vi "Stimulus XCtl Test.vi"(0 "StimChans In":T29[](array[typedef])=[{"Waveform"={"Type"=enum."Tone", "Tone"={"Frequency (kHz)"=8.0, "Phase (cycles)"=0.0, "Random phase"=TRUE}, "Pulse Train"={"Pulse width (us)"=0.0, "Pulse rate (Hz)"=0.0, "Gap (ms)"=0.0, "Polarity"=enum."POS", "PT State"={"Template"=[], "Nperiod"=0, "Index"=0, "Pulse Rate (Hz)"=0.0, "Phase (cycles)"=0.0, "Noff"=0}, "Asynch"=FALSE}, "Noise"={"Properties"={"InvFilt"=FALSE, "Aweight"=FALSE, "Seed"=0, "Tokens"=0}, "Data"={"TokenNum"=0}}, "File"={"Filename"=path "", "Signal"=[], "Channel"=0}, "FMSweep"={"Rate (oct/s)"=0.0, "Fmin (Hz)"=0.0, "Fmax (Hz)"=0.0, "Ramp (ms)"=0.0, "Linear"=FALSE}, "Chirp Train"={"Params"={"Fmin (kHz)"=4.0, "Fmax (kHz)"=64.0, "Compensate"=FALSE, "Duration (ms)"=2.0}, "Data"={"WF"=[]}}, "Complex Tone"={"Params"={"F0 (Hz)"=0.0, "Band"={"Flow (Hz)"=0.0, "Fhigh (Hz)"=0.0}, "Phase"=enum."Cosine", "Min F0 (Hz)"=0.0, "Max F0 (Hz)"=0.0, "ContinRandPhase"=FALSE, "Max peak factor"=inf, "Max mod depth"=2.0, "MinHarmNum"=0, "MaxHarmNum"=0, "Level Mode"=enum."per component"}, "Data"={"Ncomp"=0, "MinHarm"=0, "Phase"=[], "Amplitude"=[], "Npts/frame"=0, "Last F0"=0.0, "Fmin"=0.0, "Fmax"=0.0, "Lslope"=0.0, "randphase"=FALSE, "overall rms"=FALSE}}, "FM"={"Carrier (kHz)"=0.0, "ModRate (Hz)"=0.0, "Depth (Hz)"=0.0, "Phase (cycles)"=0.0}, "Vowel"={"Freqs"="", "Set level"=enum."Total", "Freq"=[], "weights"=[]}}, "Filter"={"Type"=enum."OFF", "CF (kHz)"=0.0, "BW (kHz)"=0.0, "Cascade"=FALSE, "Quadrature"=FALSE, "Scale Factor"=0.0, "Stages"=[], "Class"=enum."Elliptic", "Order"=0, "BWUnits"=enum."Linear"}, "Burst"={"Active"=FALSE, "Delay (ms)"=0.0, "Duration (ms)"=0.0, "Ramp (ms)"=0.0, "Rate (Hz)"=0.0, "Trepeat (ms)"=0.0, "Repeat"=FALSE}, "Level"={"Level"=0.0, "Units"=enum."dB atten", "Max"=0.0, "Data"={"Multiplier"=0.0, "Cal File"=path "", "Cal"={"Freq (Hz)"=[], "Mag (dB SPL)"=[], "Phase (deg)"=[]}, "audiogram"=path ""}}, "Name"="Ch1", "Advanced"={"AltPol"=FALSE, "Var"="", "Expr"=""}, "SAM"={"Active"=FALSE, "Frequency (Hz)"=0.0, "Depth"=0.0, "Init Phase (cycles)"=0.0, "phase (degrees)"=0.0, "Asynch"=FALSE}, "Destination"={"Name"="Right", "Num"=0}}, {"Waveform"={"Type"=enum."Tone", "Tone"={"Frequency (kHz)"=8.0, "Phase (cycles)"=0.0, "Random phase"=FALSE}, "Pulse Train"={"Pulse width (us)"=0.0, "Pulse rate (Hz)"=0.0, "Gap (ms)"=0.0, "Polarity"=enum."POS", "PT State"={"Template"=[], "Nperiod"=0, "Index"=0, "Pulse Rate (Hz)"=0.0, "Phase (cycles)"=0.0, "Noff"=0}, "Asynch"=FALSE}, "Noise"={"Properties"={"InvFilt"=FALSE, "Aweight"=FALSE, "Seed"=0, "Tokens"=0}, "Data"={"TokenNum"=0}}, "File"={"Filename"=path "", "Signal"=[], "Channel"=0}, "FMSweep"={"Rate (oct/s)"=0.0, "Fmin (Hz)"=0.0, "Fmax (Hz)"=0.0, "Ramp (ms)"=0.0, "Linear"=FALSE}, "Chirp Train"={"Params"={"Fmin (kHz)"=4.0, "Fmax (kHz)"=64.0, "Compensate"=FALSE, "Duration (ms)"=2.0}, "Data"={"WF"=[]}}, "Complex Tone"={"Params"={"F0 (Hz)"=0.0, "Band"={"Flow (Hz)"=0.0, "Fhigh (Hz)"=0.0}, "Phase"=enum."Cosine", "Min F0 (Hz)"=0.0, "Max F0 (Hz)"=0.0, "ContinRandPhase"=FALSE, "Max peak factor"=inf, "Max mod depth"=2.0, "MinHarmNum"=0, "MaxHarmNum"=0, "Level Mode"=enum."per component"}, "Data"={"Ncomp"=0, "MinHarm"=0, "Phase"=[], "Amplitude"=[], "Npts/frame"=0, "Last F0"=0.0, "Fmin"=0.0, "Fmax"=0.0, "Lslope"=0.0, "randphase"=FALSE, "overall rms"=FALSE}}, "FM"={"Carrier (kHz)"=0.0, "ModRate (Hz)"=0.0, "Depth (Hz)"=0.0, "Phase (cycles)"=0.0}, "Vowel"={"Freqs"="", "Set level"=enum."Total", "Freq"=[], "weights"=[]}}, "Filter"={"Type"=enum."OFF", "CF (kHz)"=0.0, "BW (kHz)"=0.0, "Cascade"=FALSE, "Quadrature"=FALSE, "Scale Factor"=0.0, "Stages"=[], "Class"=enum."Elliptic", "Order"=0, "BWUnits"=enum."Linear"}, "Burst"={"Active"=FALSE, "Delay (ms)"=0.0, "Duration (ms)"=0.0, "Ramp (ms)"=0.0, "Rate (Hz)"=0.0, "Trepeat (ms)"=0.0, "Repeat"=FALSE}, "Level"={"Level"=0.0, "Units"=enum."dB atten", "Max"=0.0, "Data"={"Multiplier"=0.0, "Cal File"=path "", "Cal"={"Freq (Hz)"=[], "Mag (dB SPL)"=[], "Phase (deg)"=[]}, "audiogram"=path ""}}, "Name"="Ch2", "Advanced"={"AltPol"=FALSE, "Var"="", "Expr"=""}, "SAM"={"Active"=FALSE, "Frequency (Hz)"=0.0, "Depth"=0.0, "Init Phase (cycles)"=0.0, "phase (degrees)"=0.0, "Asynch"=FALSE}, "Destination"={"Name"="Left", "Num"=1}}] {"Filter"."Stages"."IIR Filter"."Forward Coefficients" format="%.4f"; "Filter"."Stages"."IIR Filter"."Reverse Coefficients" format="%.4f"}, 1 "Folder":path=path "D:/Data/XYZ DATA/XYZ999") -> ()   [LabVIEW 2015]
uses:
  XControls/Stimulus Channel (G3)/Full Stimulus Channel Data.ctl
  XControls/Waveform XControls/Waveform (G3)/Waveform Data.ctl
  Waveform VIs/Waveform Enum (V3).ctl
  XControls/Waveform XControls/Tone (G3)/Tone.Properties.ctl
  Waveform VIs/Pulse Train VIs/Pulse Train Params.ctl
  Waveform VIs/Pulse Train VIs/Pulse Polarity.ctl
  Waveform VIs/Pulse Train VIs/PT-Continuous State.ctl
  Waveform VIs/Noise VIs/Noise (G3).ctl
  Waveform VIs/Noise VIs/Noise (G3).Properties.ctl
  Waveform VIs/Noise VIs/Noise (G3).Data.ctl
  Waveform VIs/File VIs/StimFile-Params.ctl
  Waveform VIs/FM Sweep VIs/FM Sweep Params.ctl
  Waveform VIs/Chirp Train VIs/Chirp Train.ctl
  Waveform VIs/Chirp Train VIs/Chirp Train Params.ctl
  Waveform VIs/Complex Tone VIs/CT-Params.ctl
  Waveform VIs/Complex Tone VIs/CT-Phase Enum.ctl
  Waveform VIs/Complex Tone VIs/CT-Runtime Data.ctl
  XControls/Waveform XControls/FM Tone/Data.ctl
  XControls/Waveform XControls/Vowel/Vowel.Properties.ctl
  XControls/Filter (G3)/Filter Data.ctl
  XControls/Filter (G3)/Filter Type.ctl
  Filter VIs/Filter-Bandwidth Units.ctl
  Controls/Burst XCtl/Burst Data.ctl
  XControls/Level (G3)/Level Data.ctl
  XControls/Level (G3)/Level Units (G3).ctl
  XControls/Advanced Options (G3)/Advanced Options (G3).ctl
  Modulation VIs/SAM VIs/SAM Params.ctl
  Typedefs/Destination.ctl
  XControls/Stimulus Channel (G3)/Stimulus Channel (G3).xctl
  XControls/Waveform XControls/Waveform (G3)/Waveform (G3).xctl
  XControls/Filter (G3)/Filter (G3).xctl
  Controls/Burst XCtl/Burst Control.xctl
  XControls/Level (G3)/Level (G3).xctl
  XControls/Advanced Options (G3)/Advanced Options (G3).xctl
  XControls/Waveform XControls/Tone (G3)/Tone (G3).xctl
  XControls/Waveform XControls/FM Tone/FM Tone.xctl
  XControls/Waveform XControls/Vowel/Vowel.xctl
panel:
  in  "Drag from":i32
  in  "StimChan":T28(xcontrol)
  out "exit signal":bool
  in  "Delete":bool
  in  "Insert":bool
  in  "Apply":bool
  in  "Channels":i32[](listbox)
  # "Right Primary"
  # "Right Primary"
  # "Laser1"
  # "Right Primary"
  # "Right Primary"
  # "Laser2"
  # "Right Primary"
  # "Shutter"
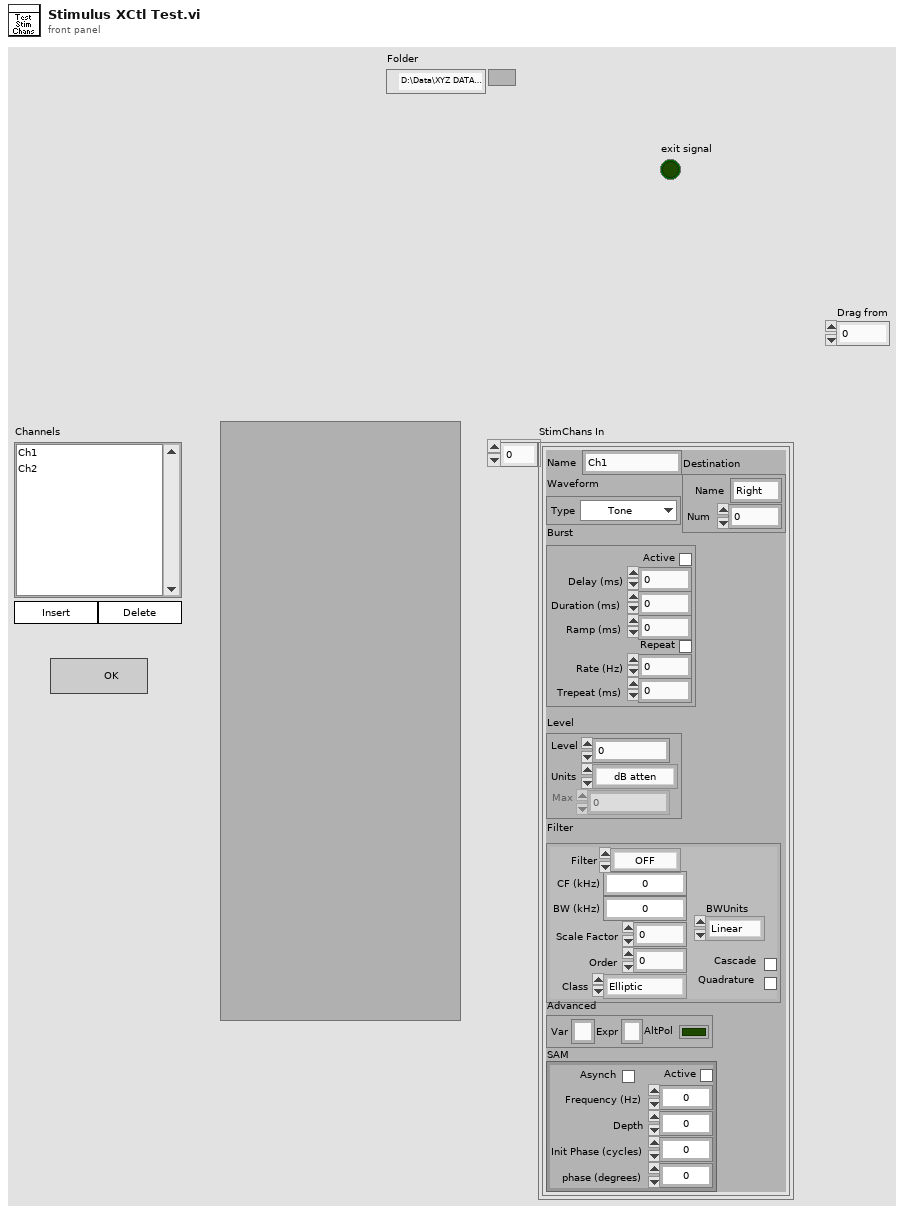
[diagram p1: front panel]
types:
  T1 = typedef "Waveform (G3).xctl/Waveform Data.ctl" = cluster{"Type":T2, "Tone":T3, "Pulse Train":T4, "Noise":T7, "File":T10, "FMSweep":T11, "Chirp Train":T12, "Complex Tone":cluster{"Params":T14, "Data":T16}, "FM":T17, "Vowel":T18}
  T2 = typedef "Waveform Enum (V3).ctl" = enum16{"OFF", "Tone", "Noise", "Pulse Train", "File", "FM Sweep", "Chirp Train", "Complex Tone", "FM Tone", "Vowel"}
  T3 = typedef "Tone (G3).xctl/Tone.Properties.ctl" = cluster{"Frequency (kHz)":dbl, "Phase (cycles)":dbl, "Random phase":bool}
  T4 = typedef "Pulse Train Params.ctl" = cluster{"Pulse width (us)":dbl, "Pulse rate (Hz)":dbl, "Gap (ms)":dbl, "Polarity":T5, "PT State":T6, "Asynch":bool}
  T5 = typedef "Pulse Polarity.ctl" = enum16{"POS", "NEG", "POS-NEG", "NEG-POS"}
  T6 = typedef "PT-Continuous State.ctl" = cluster{"Template":dbl[], "Nperiod":i32, "Index":i32, "Pulse Rate (Hz)":dbl, "Phase (cycles)":dbl, "Noff":i32}
  T7 = typedef "Noise (G3).ctl" = cluster{"Properties":T8, "Data":T9}
  T8 = typedef "Noise (G3).Properties.ctl" = cluster{"InvFilt":bool, "Aweight":bool, "Seed":i32, "Tokens":i32}
  T9 = typedef "Noise (G3).Data.ctl" = cluster{"TokenNum":i32}
  T10 = typedef "StimFile-Params.ctl" = cluster{"Filename":path, "Signal":dbl[], "Channel":i32}
  T11 = typedef "FM Sweep Params.ctl" = cluster{"Rate (oct/s)":dbl, "Fmin (Hz)":dbl, "Fmax (Hz)":dbl, "Ramp (ms)":dbl, "Linear":bool}
  T12 = typedef "Chirp Train.ctl" = cluster{"Params":T13, "Data":cluster{"WF":dbl[]}}
  T13 = typedef "Chirp Train Params.ctl" = cluster{"Fmin (kHz)":dbl, "Fmax (kHz)":dbl, "Compensate":bool, "Duration (ms)":dbl}
  T14 = typedef "CT-Params.ctl" = cluster{"F0 (Hz)":dbl, "Band":cluster{"Flow (Hz)":dbl, "Fhigh (Hz)":dbl}, "Phase":T15, "Min F0 (Hz)":dbl, "Max F0 (Hz)":dbl, "ContinRandPhase":bool, "Max peak factor":dbl, "Max mod depth":dbl, "MinHarmNum":i32, "MaxHarmNum":i32, "Level Mode":enum16{"per component", "overall rms"}}
  T15 = typedef "CT-Phase Enum.ctl" = enum16{"Cosine", "Random", "Alternating"}
  T16 = typedef "CT-Runtime Data.ctl" = cluster{"Ncomp":i32, "MinHarm":i32, "Phase":dbl[], "Amplitude":dbl[], "Npts/frame":i32, "Last F0":dbl, "Fmin":dbl, "Fmax":dbl, "Lslope":dbl, "randphase":bool, "overall rms":bool}
  T17 = typedef "FM Tone.xctl/Data.ctl" = cluster{"Carrier (kHz)":dbl, "ModRate (Hz)":dbl, "Depth (Hz)":dbl, "Phase (cycles)":dbl}
  T18 = typedef "Vowel.xctl/Vowel.Properties.ctl" = cluster{"Freqs":string, "Set level":enum16{"Total", "Per component"}, "Freq":dbl[], "weights":dbl[]}
  T19 = typedef "Filter (G3).xctl/Filter Data.ctl" = cluster{"Type":T20, "CF (kHz)":dbl, "BW (kHz)":dbl, "Cascade":bool, "Quadrature":bool, "Scale Factor":dbl, "Stages":cluster{"IIR Filter":cluster{"filter structure":enum32{"IIR 2nd Order", "IIR 4th Order"}, "Reverse Coefficients":dbl[], "Forward Coefficients":dbl[]}, "State":dbl[]}[], "Class":enum16{"Elliptic", "Butterworth"}, "Order":i32, "BWUnits":T21}
  T20 = typedef "Filter (G3).xctl/Filter Type.ctl" = enum16{"OFF", "Lowpass", "Highpass", "Bandpass", "Bandstop"}
  T21 = typedef "Filter-Bandwidth Units.ctl" = enum16{"Linear", "Octaves", "Min-Max"}
  T22 = typedef "Burst Control.xctl/Burst Data.ctl" = cluster{"Active":bool, "Delay (ms)":dbl, "Duration (ms)":dbl, "Ramp (ms)":dbl, "Rate (Hz)":dbl, "Trepeat (ms)":dbl, "Repeat":bool}
  T23 = typedef "Level (G3).xctl/Level Data.ctl" = cluster{"Level":dbl, "Units":T24, "Max":dbl, "Data":cluster{"Multiplier":dbl, "Cal File":path, "Cal":cluster{"Freq (Hz)":dbl[], "Mag (dB SPL)":dbl[], "Phase (deg)":dbl[]}, "audiogram":path}}
  T24 = typedef "Level (G3).xctl/Level Units (G3).ctl" = enum16{"dB atten", "dB SPL", "dB re 1 Vrms", "dB V/Hz½", "dB SL", "mW", "Volts"}
  T25 = typedef "Advanced Options (G3).xctl/Advanced Options (G3).ctl" = cluster{"AltPol":bool, "Var":string, "Expr":string}
  T26 = typedef "SAM Params.ctl" = cluster{"Active":bool, "Frequency (Hz)":dbl, "Depth":dbl, "Init Phase (cycles)":dbl, "phase (degrees)":dbl, "Asynch":bool}
  T27 = typedef "Destination.ctl" = cluster{"Name":string, "Num":i32}
  T28 = cluster{"Waveform":T1, "Filter":T19, "Burst":T22, "Level":T23, "Name":string, "Advanced":T25, "SAM":T26, "Destination":T27}
  T29 = typedef "Stimulus Channel (G3).xctl/Full Stimulus Channel Data.ctl" = cluster{"Waveform":T1, "Filter":T19, "Burst":T22, "Level":T23, "Name":string, "Advanced":T25, "SAM":T26, "Destination":T27}
  T30 = typedef "Endpoint-Spec.ctl" = cluster{"Name":string, "Modality":T31, "Laterality":T32, "CalFile":path, "Audiogram":path, "reuse cal?":bool}
  T31 = typedef "Endpoint-Modality.ctl" = enum16{"Unspecified", "Acoustic", "Electric", "Optical"}
  T32 = typedef "Endpoint-Laterality.ctl" = enum16{"N/A", "Right", "Left"}
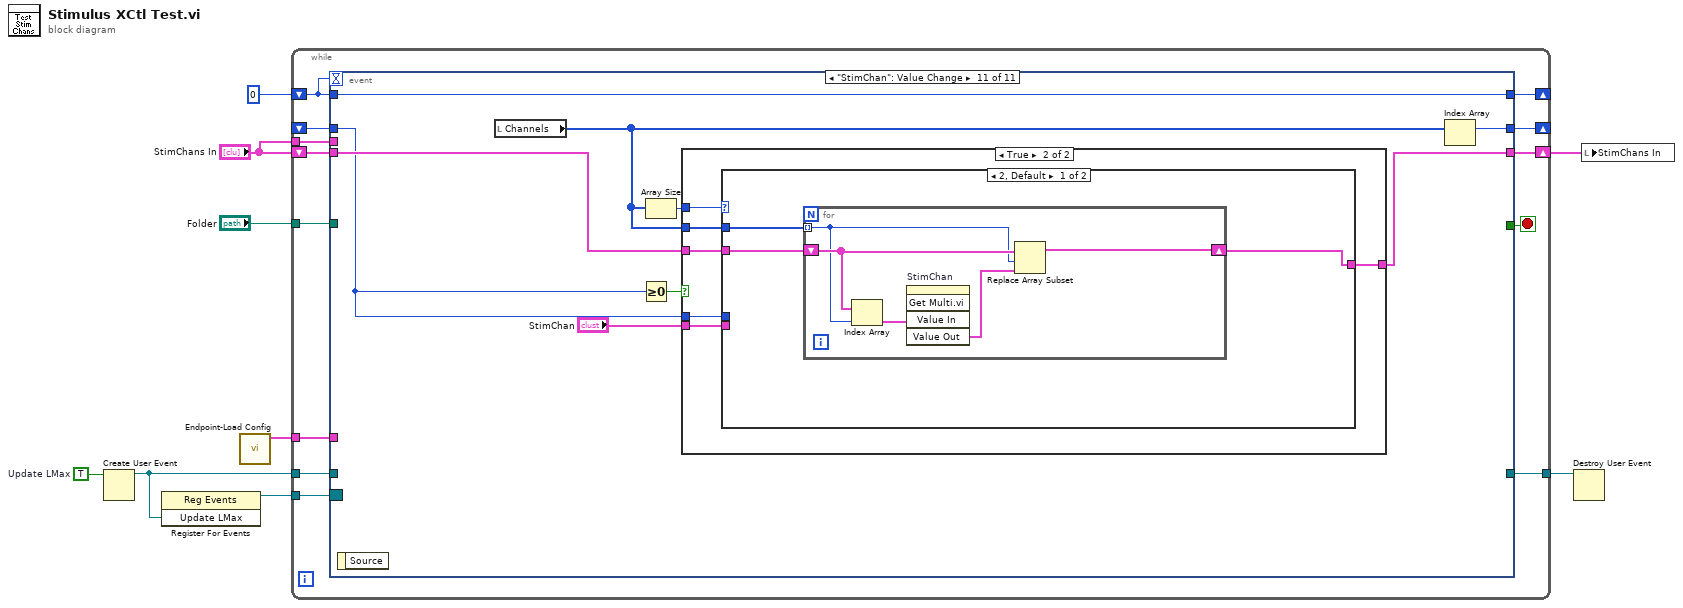
[diagram p0: block diagram]
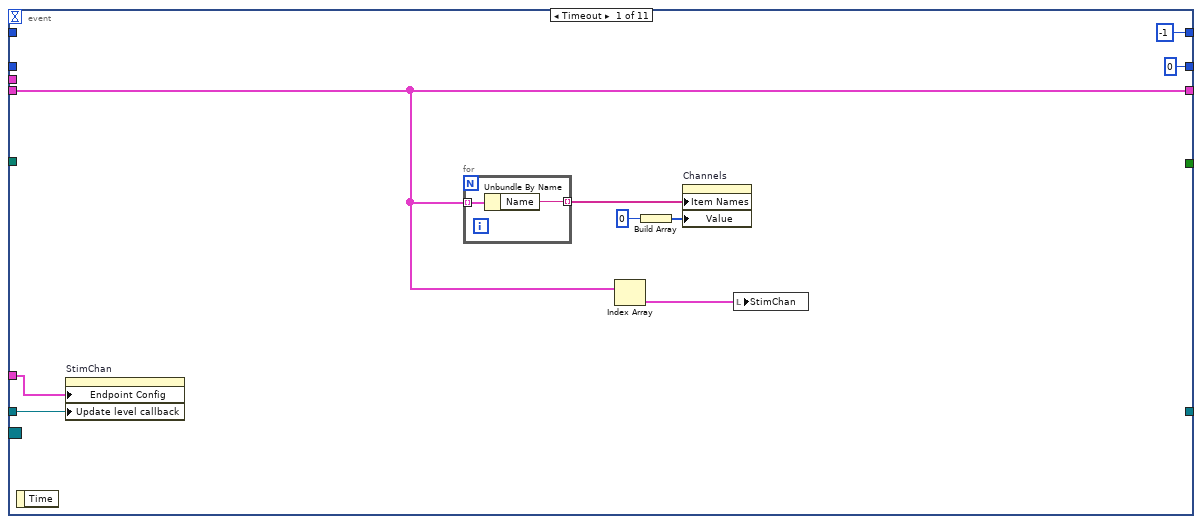
[diagram p2: hidden frame]
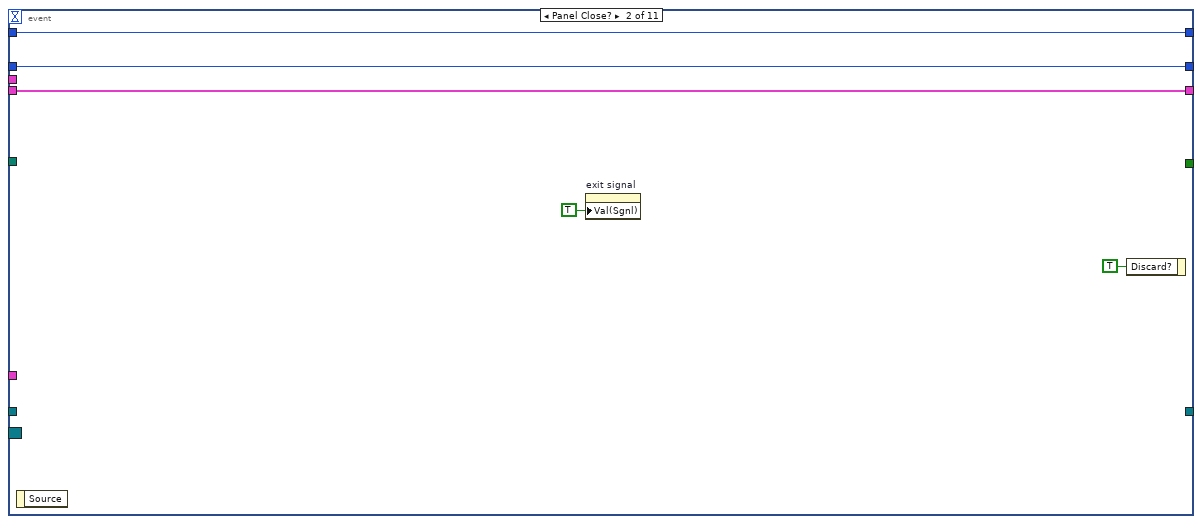
[diagram p3: hidden frame]
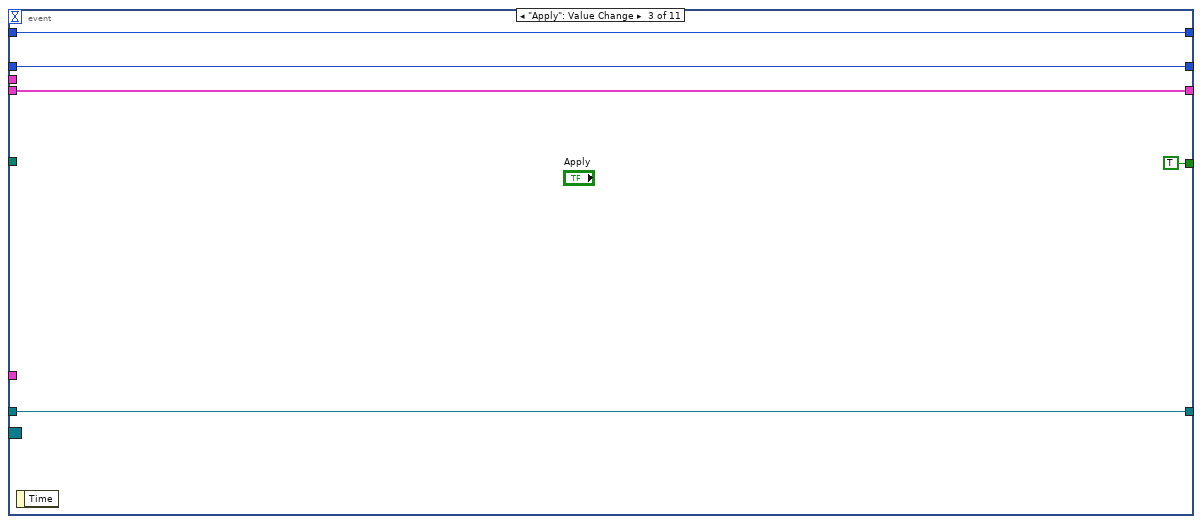
[diagram p4: hidden frame]
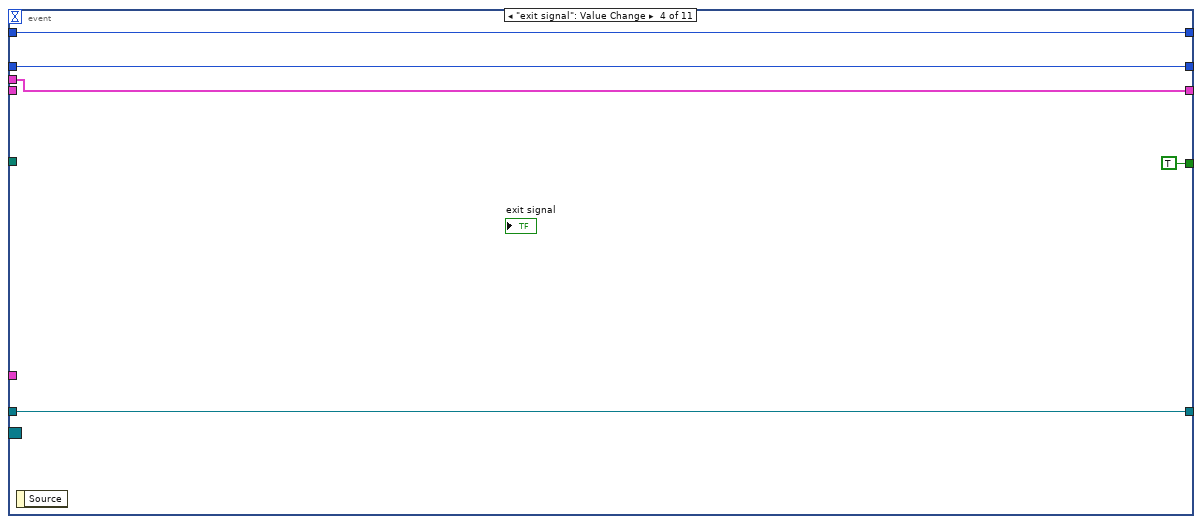
[diagram p5: hidden frame]
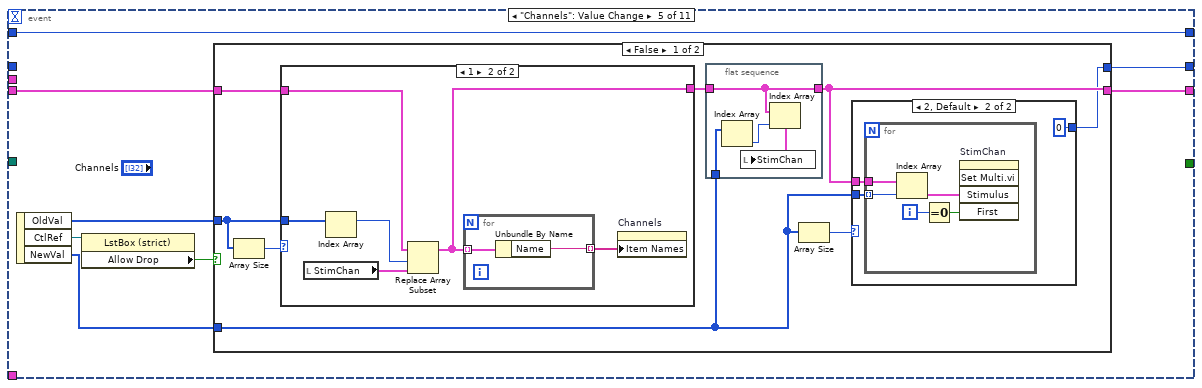
[diagram p6: hidden frame]
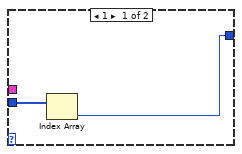
[diagram p7: hidden frame]
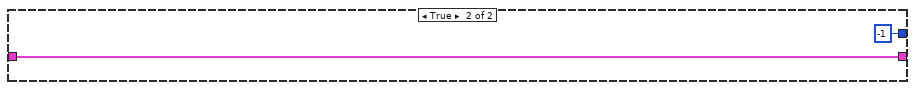
[diagram p9: hidden frame]
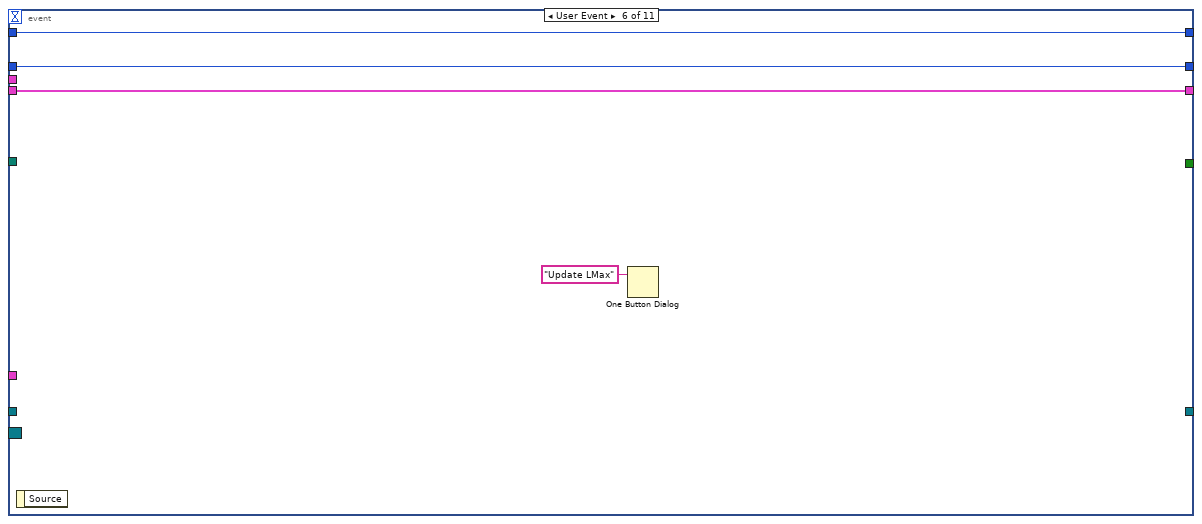
[diagram p10: hidden frame]
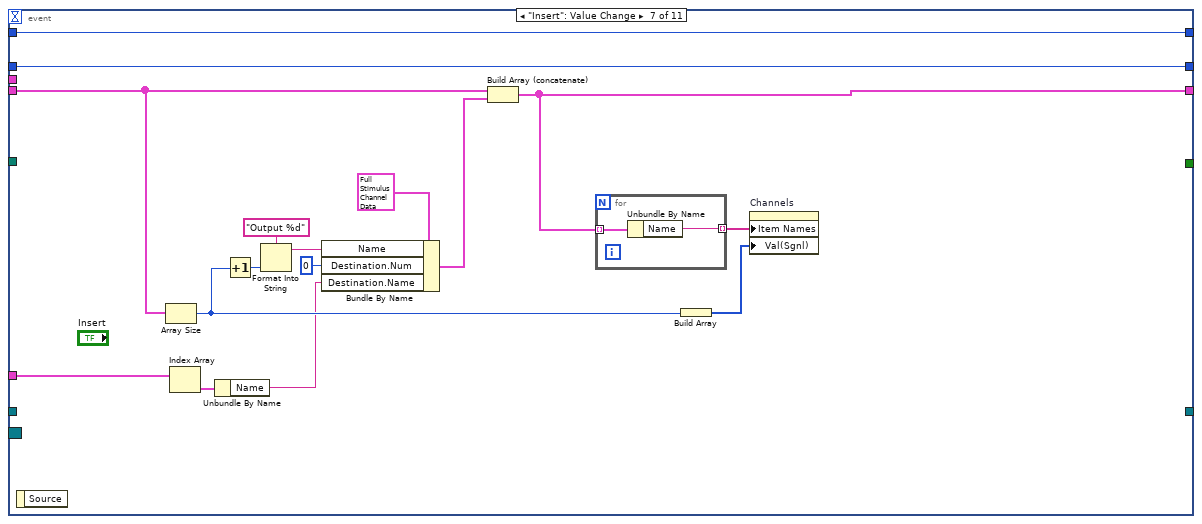
[diagram p11: hidden frame]
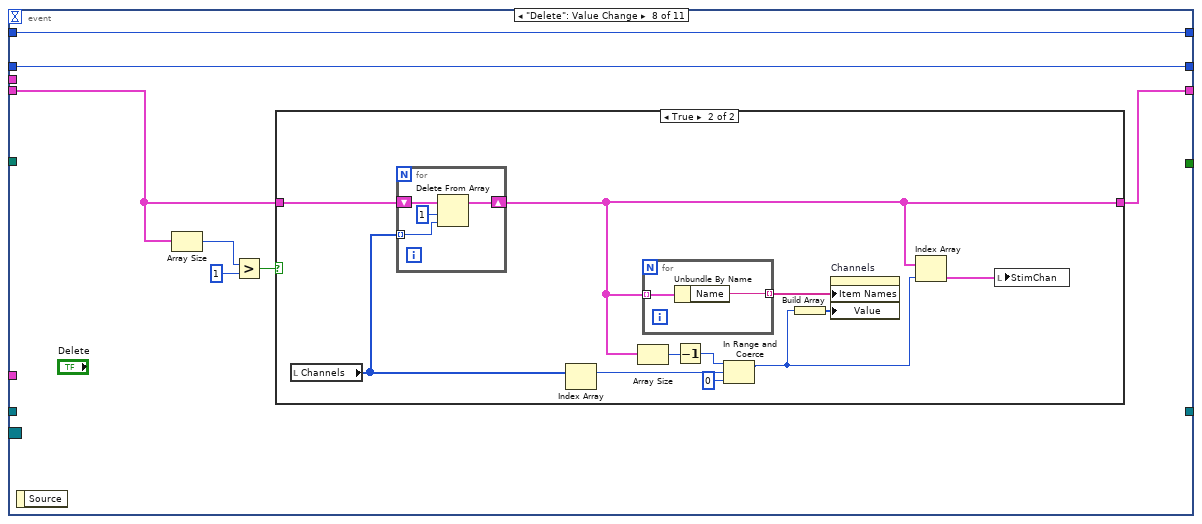
[diagram p12: hidden frame]
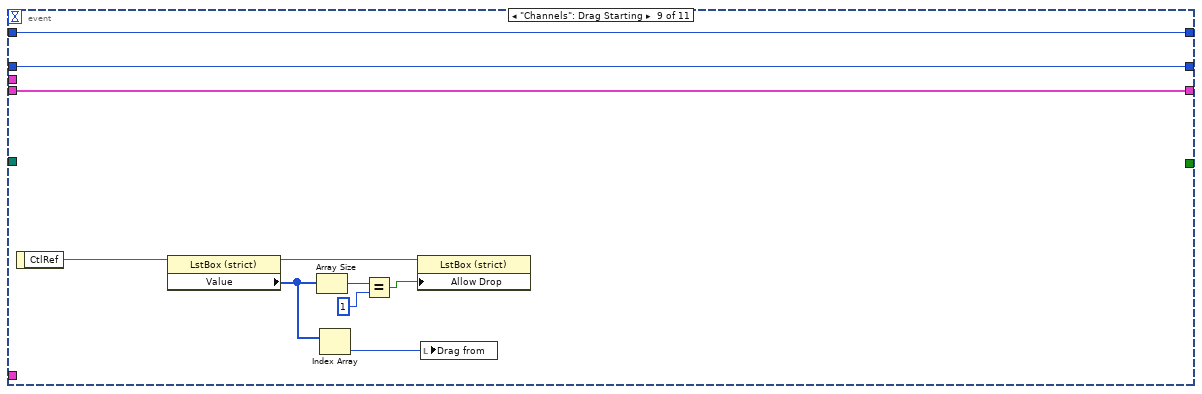
[diagram p14: hidden frame]
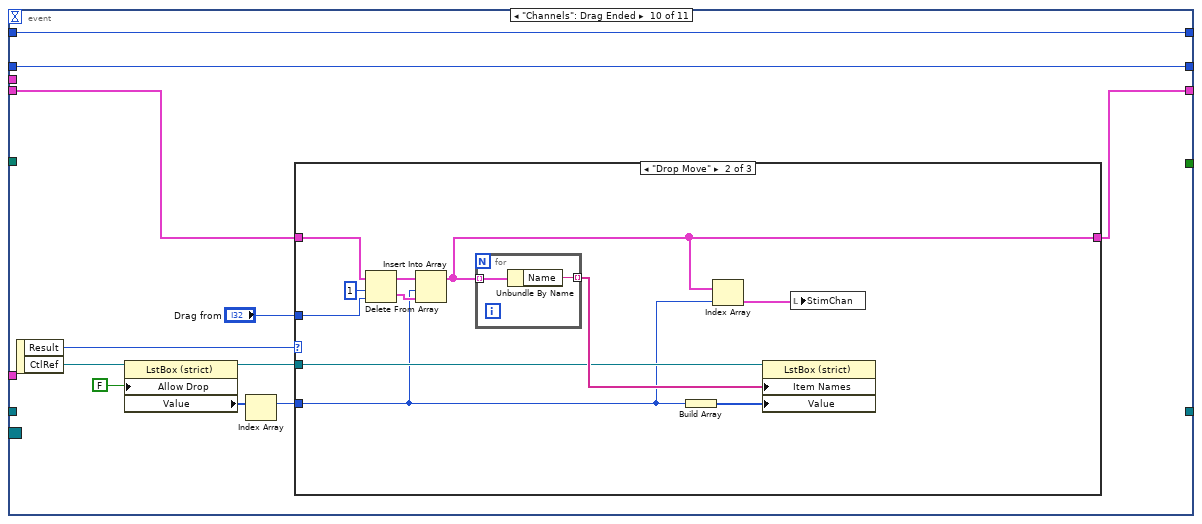
[diagram p15: hidden frame]
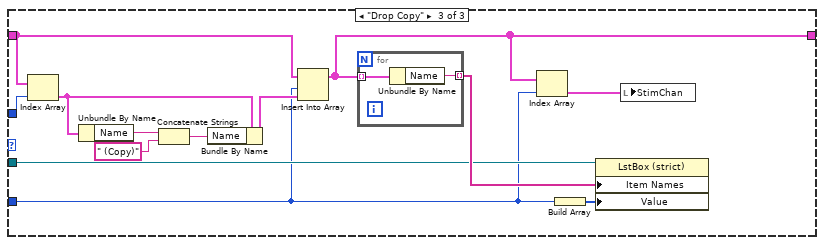
[diagram p17: hidden frame]
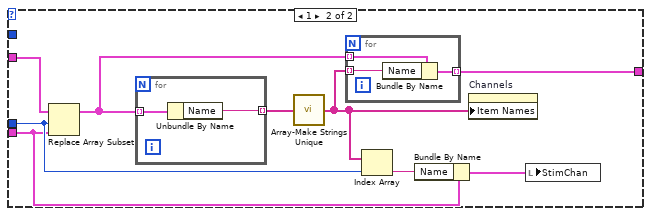
[diagram p19: hidden frame]
diagram:
  w7 = TRUE  # Update LMax
  n1 = Create User Event(user event datatype=w7) -> (user event=w5:refnum<user-event>)  [unwired: 1 in, 1 out]
  n2 = register-events(w5) -> (reference out=w6:refnum<event-registration>)  [unwired: 2 in, 1 out]
  n3 = call "Endpoint-Load Config.vi"() -> ("Endpoint Config"=w2:T30[])  [unwired: 10 in, 1 out]
  n4 = while {
    shift-right: [w22] -> _
    shift-left: 0 -> [w20]
    shift-right: [w18] -> w1
    shift-left: "StimChans In" -> [w19]
    tunnel: "StimChans In" -> [w17]
    tunnel: w6 -> [w16]
    tunnel: w5 -> [w15]
    tunnel: w2 -> [w14]
    tunnel: "Folder" -> [w13]
    shift-right: [w12] -> _
    shift-left: _ -> [w11]
    tunnel: [w10] -> w3
    stop <- w21 stop-if-true
    n5 = event shown="[10] \"StimChan\": Value Change" {
      selector: w16 -> [_ _ _ _ _ _ _ _ _ _ _]
      dyn-events: _ -> [_ _ _ _ _ _ _ _ _ _ _]
      timeout: w20 -> [_ _ _ _ _ _ _ _ _ _ _]
      tunnel: [-1 w38 w42 w47 w56 w93 w109 w118 w146 w157 w195] -> w22
      tunnel: [_ _ TRUE TRUE _ _ _ _ _ _ _] -> w21
      tunnel: w20 -> [_ w38 w42 w47 w56 w93 w109 w118 w146 w157 w195]
      tunnel: w19 -> [w27 w37 w41 _ w54 w92 w108 w115 w145 w153 w194]
      tunnel: [w27 w37 w41 w46 w53 w92 w102 w114 w145 w151 w193] -> w18
      tunnel: w17 -> [_ _ _ w46 _ _ _ _ _ _ _]
      tunnel: w15 -> [w30 _ w39 w44 _ _ _ _ _ _ _]
      tunnel: w14 -> [w31 _ _ _ _ _ w98 _ _ _ _]
      tunnel: w13 -> [_ _ _ _ _ _ _ _ _ _ _]
      tunnel: [0 ("Channels") w34 w40 w45 w49 w91 w99 w112 w144 w148 w189] -> w12
      tunnel: w11 -> [_ w34 w40 w45 _ w91 w99 w112 w144 w148 w190]
      tunnel: [_ _ w39 w44 _ _ _ _ _ _ _] -> w10
      event Timeout {
        n6 = event-data() -> ()  [unwired: 1 in, 1 out]
        n7 = property on="StimChan" class="Stimulus Channel (G3) (strict)"("Endpoint Config"=w31, "Update level callback"=w30) -> ()  [unwired: 2 in, 2 out]
        n8 = for {
          tunnel: w27 -> [w33] mode=indexing
          tunnel: [w32] -> w25 mode=indexing
          n9 = Unbundle By Name(w33) -> ("Name"=w32:string)
        }
        n10 = Index Array(array=w27) -> (element=w23:T29)  [unwired: 1 in]
        n11 = Build Array(0) -> (w24:i32[])
        n12 = property on="Channels" class="LstBox (strict)"("Item Names"=w25, "Value"=w24) -> ()  [unwired: 2 in, 2 out]
        n13 = local write "StimChan"(w23) -> ()
      }
      event Panel Close? {
        n14 = event-data() -> ()  [unwired: 1 in, 1 out]
        n15 = property on="exit signal" class="Bool (strict)"("Val(Sgnl)"=TRUE ("Value (Signaling)")) -> ()  [unwired: 2 in, 2 out]
        n16 = event-data("Discard?"=TRUE) -> ()  [unwired: 1 in, 1 out]
      }
      event "Apply": Value Change {
        n17 = event-data() -> ()  [unwired: 1 in, 1 out]
      }
      event "exit signal": Value Change {
        n18 = event-data() -> ()  [unwired: 1 in, 1 out]
      }
      event "Channels": Value Change {
        n19 = event-data() -> ("OldVal"=w55:i32[], "CtlRef"=w52:refnum<vi>, "NewVal"=w50:i32[])  [unwired: 1 in]
        n20 = property class="LstBox (strict)"(reference=w52) -> ("Allow Drop"=w51:bool)  [unwired: 1 in, 2 out]
        n21 = case shown="False" w51 {
          tunnel: w55 -> [w62 _]
          tunnel: w54 -> [w61 w89]
          tunnel: [w58 w89] -> w53
          tunnel: w50 -> [w60 _]
          tunnel: [w57 -1 ("Channels")] -> w49
          frame False {
            n22 = Array Size(array=w62) -> (size(s)=w64:i32)
            n23 = case shown="1" w64 {
              tunnel: w62 -> [_ w85]
              tunnel: [w79 w81] -> w59
              tunnel: w61 -> [w79 w80]
              frame 2, Default {
              }
              frame 1 {
                n24 = local read "StimChan"() -> (w84:T28)
                n25 = Index Array(array=w85) -> (element=w83:i32)  [unwired: 1 in]
                n26 = Replace Array Subset(array=w80, new element=w84, index=w83) -> (w81:T29[])
                n27 = for {
                  tunnel: w81 -> [w87] mode=indexing
                  tunnel: [w86] -> w82 mode=indexing
                  n28 = Unbundle By Name(w87) -> ("Name"=w86:string)
                }
                n29 = property on="Channels" class="LstBox (strict)"("Item Names"=w82) -> ()  [unwired: 2 in, 2 out]
              }
            }
            n30 = flat-sequence {
              tunnel: w60 -> [w66]
              tunnel: w59 -> [w65]
              tunnel: [w65] -> w58
              frame #0 {
                n31 = Index Array(array=w66) -> (element=w67:i32)  [unwired: 1 in]
                n32 = Index Array(array=w65, index=w67) -> (element=w68:T29)
                n33 = local write "StimChan"(w68) -> ()
              }
            }
            n34 = Array Size(array=w60) -> (size(s)=w63:i32)
            n35 = case shown="2, Default" w63 {
              tunnel: w58 -> [_ w73]
              tunnel: w60 -> [w70 w72]
              tunnel: [w69 0] -> w57
              frame 1 {
                n36 = Index Array(array=w70) -> (element=w69:i32)  [unwired: 1 in]
              }
              frame 2, Default {
                n37 = for {
                  tunnel: w73 -> [w78]
                  tunnel: w72 -> [w77] mode=indexing
                  i -> [w74]
                  n38 = Index Array(array=w78, index=w77) -> (element=w76:T29)
                  n39 = Equal To 0?(x=w74) -> (x = 0?=w75:bool)
                  n40 = invoke on="StimChan" class="Stimulus Channel (G3) (strict)" method="Set Multi.vi"("Stimulus"=w76, "First"=w75) -> ()  [unwired: 3 in, 5 out]
                }
              }
            }
          }
          frame True {
          }
        }
      }
      event User Event {
        n41 = event-data() -> ()  [unwired: 1 in, 1 out]
        n42 = One Button Dialog(message="Update LMax") -> ()  [unwired: 1 in, 1 out]
      }
      event "Insert": Value Change {
        n43 = event-data() -> ()  [unwired: 1 in, 1 out]
        n44 = Array Size(array=w108) -> (size(s)=w100:i32)
        n45 = Index Array(array=w98) -> (element=w97:T30)  [unwired: 1 in]
        n46 = Unbundle By Name(w97) -> ("Name"=w96:string)
        n47 = Increment(x=w100) -> (x+1=w105:i32)
        n48 = Format Into String(format string="Output %d", w105) -> (resulting string=w104:string)  [unwired: 2 in, 1 out]
        n49 = Bundle By Name(cluster=T29 {"Waveform"={"Type"=enum."Tone", "Tone"={"Frequency (kHz)"=0.0, "Phase (cycles)"=0.0, "Random phase"=FALSE}, "Pulse Train"={"Pulse width (us)"=0.0, "Pulse rate (Hz)"=0.0, "Gap (ms)"=0.0, "Polarity"=enum."POS", "PT State"={"Template"=[], "Nperiod"=0, "Index"=0, "Pulse Rate (Hz)"=0.0, "Phase (cycles)"=0.0, "Noff"=0}, "Asynch"=FALSE}, "Noise"={"Properties"={"InvFilt"=FALSE, "Aweight"=FALSE, "Seed"=0, "Tokens"=0}, "Data"={"TokenNum"=0}}, "File"={"Filename"=path "", "Signal"=[], "Channel"=0}, "FMSweep"={"Rate (oct/s)"=0.0, "Fmin (Hz)"=0.0, "Fmax (Hz)"=0.0, "Ramp (ms)"=0.0, "Linear"=FALSE}, "Chirp Train"={"Params"={"Fmin (kHz)"=4.0, "Fmax (kHz)"=64.0, "Compensate"=FALSE, "Duration (ms)"=2.0}, "Data"={"WF"=[]}}, "Complex Tone"={"Params"={"F0 (Hz)"=0.0, "Band"={"Flow (Hz)"=0.0, "Fhigh (Hz)"=0.0}, "Phase"=enum."Cosine", "Min F0 (Hz)"=0.0, "Max F0 (Hz)"=0.0, "ContinRandPhase"=FALSE, "Max peak factor"=inf, "Max mod depth"=2.0, "MinHarmNum"=0, "MaxHarmNum"=0, "Level Mode"=enum."per component"}, "Data"={"Ncomp"=0, "MinHarm"=0, "Phase"=[], "Amplitude"=[], "Npts/frame"=0, "Last F0"=0.0, "Fmin"=0.0, "Fmax"=0.0, "Lslope"=0.0, "randphase"=FALSE, "overall rms"=FALSE}}, "FM"={"Carrier (kHz)"=0.0, "ModRate (Hz)"=0.0, "Depth (Hz)"=0.0, "Phase (cycles)"=0.0}, "Vowel"={"Freqs"="", "Set level"=enum."Total", "Freq"=[], "weights"=[]}}, "Filter"={"Type"=enum."Lowpass", "CF (kHz)"=0.0, "BW (kHz)"=0.0, "Cascade"=FALSE, "Quadrature"=FALSE, "Scale Factor"=0.0, "Stages"=[], "Class"=enum."Elliptic", "Order"=0, "BWUnits"=enum."Linear"}, "Burst"={"Active"=FALSE, "Delay (ms)"=0.0, "Duration (ms)"=0.0, "Ramp (ms)"=0.0, "Rate (Hz)"=0.0, "Trepeat (ms)"=0.0, "Repeat"=FALSE}, "Level"={"Level"=0.0, "Units"=enum."dB atten", "Max"=0.0, "Data"={"Multiplier"=0.0, "Cal File"=path "", "Cal"={"Freq (Hz)"=[], "Mag (dB SPL)"=[], "Phase (deg)"=[]}, "audiogram"=path ""}}, "Name"="", "Advanced"={"AltPol"=FALSE, "Var"="", "Expr"=""}, "SAM"={"Active"=FALSE, "Frequency (Hz)"=0.0, "Depth"=0.0, "Init Phase (cycles)"=0.0, "phase (degrees)"=0.0, "Asynch"=FALSE}, "Destination"={"Name"="", "Num"=0}} ("Stimulus"), "Name"=w104, "Destination.Num"=0, "Destination.Name"=w96) -> (w103:T29)
        n50 = Build Array (concatenate)(w108, w103) -> (w102:T29[])
        n51 = for {
          tunnel: w102 -> [w111] mode=indexing
          tunnel: [w110] -> w101 mode=indexing
          n52 = Unbundle By Name(w111) -> ("Name"=w110:string)
        }
        n53 = Build Array(w100) -> (w94:i32[])
        n54 = property on="Channels" class="LstBox (strict)"("Item Names"=w101, "Val(Sgnl)"=w94) -> ()  [unwired: 2 in, 2 out]
      }
      event "Delete": Value Change {
        n55 = event-data() -> ()  [unwired: 1 in, 1 out]
        n56 = Array Size(array=w115) -> (size(s)=w113:i32)
        n57 = Greater?(x=w113, y=1) -> (0:w116:bool)
        n58 = case shown="True" w116 {
          tunnel: w115 -> [w119 w130]
          tunnel: [w119 w123] -> w114
          frame False {
          }
          frame True {
            n59 = local read "Channels"() -> (w129:i32[])
            n60 = for {
              tunnel: w129 -> [w134] mode=indexing
              shift-right: [w133] -> w123
              shift-left: w130 -> [w136]
              n61 = Delete From Array(array=w136, length=1, index=w134) -> (array with subset deleted=w133:T29[])  [unwired: 1 out]
            }
            n62 = Index Array(array=w129) -> (element=w122:i32)  [unwired: 1 in]
            n63 = Array Size(array=w123) -> (size(s)=w128:i32)
            n64 = for {
              tunnel: w123 -> [w132] mode=indexing
              tunnel: [w131] -> w124 mode=indexing
              n65 = Unbundle By Name(w132) -> ("Name"=w131:string)
            }
            n66 = Decrement(x=w128) -> (x-1=w127:i32)
            n67 = In Range and Coerce(upper limit=w127, x=w122, lower limit=0) -> (coerced(x)=w121:i32)  [unwired: 1 out]
            n68 = Build Array(w121) -> (w120:i32[])
            n69 = property on="Channels" class="LstBox (strict)"("Item Names"=w124, "Value"=w120) -> ()  [unwired: 2 in, 2 out]
            n70 = Index Array(array=w123, index=w121) -> (element=w125:T29)
            n71 = local write "StimChan"(w125) -> ()
          }
        }
      }
      event "Channels": Drag Starting {
        n72 = event-data() -> ("CtlRef"=w143:refnum<vi>)  [unwired: 1 in]
        n73 = property class="LstBox (strict)"(reference=w143) -> (reference out=w142:refnum<vi>, "Value"=w138:i32[])  [unwired: 1 in, 1 out]
        n74 = Array Size(array=w138) -> (size(s)=w141:i32)
        n75 = Index Array(array=w138) -> (element=w137:i32)  [unwired: 1 in]
        n76 = Equal?(x=w141, y=1) -> (x = y?=w139:bool)
        n77 = property class="LstBox (strict)"(reference=w142, "Allow Drop"=w139) -> ()  [unwired: 1 in, 2 out]
        n78 = local write "Drag from"(w137) -> ()
      }
      event "Channels": Drag Ended {
        n79 = event-data() -> ("Result"=w154:enum16{"Drop Cancel", "Drop Move", "Drop Copy"}, "CtlRef"=w155:refnum<vi>)  [unwired: 1 in]
        n80 = property class="LstBox (strict)"(reference=w155, "Allow Drop"=FALSE ("Drag/Drop:Allow Dropping")) -> (reference out=w150:refnum<vi>, "Value"=w149:i32[])  [unwired: 1 in, 1 out]
        n81 = Index Array(array=w149) -> (element=w147:i32)  [unwired: 1 in]
        n82 = case shown="\"Drop Move\"" w154 {
          tunnel: w153 -> [w158 w166 w182]
          tunnel: "Drag from" -> [_ w165 w181]
          tunnel: [w158 w162 w175] -> w151
          tunnel: w150 -> [_ w163 w183]
          tunnel: w147 -> [_ w160 w173]
          frame "Drop Cancel", Default {
          }
          frame "Drop Move" {
            n83 = Delete From Array(array=w166, length=1, index=w165) -> (deleted portion=w169:T29[], array with subset deleted=w167:T29[])
            n84 = Insert Into Array(array=w167, index=w160, new element=w169) -> (w162:T29[])
            n85 = for {
              tunnel: [w171] -> w164 mode=indexing
              tunnel: w162 -> [w170] mode=indexing
              n86 = Unbundle By Name(w170) -> ("Name"=w171:string)
            }
            n87 = Build Array(w160) -> (w159:i32[])
            n88 = Index Array(array=w162, index=w160) -> (element=w161:T29)
            n89 = property on="Property Node" class="LstBox (strict)"(reference=w163, "Item Names"=w164, "Value"=w159) -> ()  [unwired: 1 in, 2 out]
            n90 = local write "StimChan"(w161) -> ()
          }
          frame "Drop Copy" {
            n91 = Index Array(array=w182, index=w181) -> (element=w180:T29)
            n92 = Unbundle By Name(w180) -> ("Name"=w179:string)
            n93 = Concatenate Strings(w179, " (Copy)" ("string")) -> (w176:string)
            n94 = Bundle By Name(cluster=w180, "Name"=w176) -> (w177:T29)
            n95 = Insert Into Array(array=w182, index=w173, new element=w177) -> (w175:T29[])
            n96 = for {
              tunnel: [w186] -> w184 mode=indexing
              tunnel: w175 -> [w185] mode=indexing
              n97 = Unbundle By Name(w185) -> ("Name"=w186:string)
            }
            n98 = Index Array(array=w175, index=w173) -> (element=w174:T29)
            n99 = Build Array(w173) -> (w172:i32[])
            n100 = property on="Property Node" class="LstBox (strict)"(reference=w183, "Item Names"=w184, "Value"=w172) -> ()  [unwired: 1 in, 2 out]
            n101 = local write "StimChan"(w174) -> ()
          }
        }
      }
      event "StimChan": Value Change {
        n102 = event-data() -> ()  [unwired: 1 in, 1 out]
        n103 = local read "Channels"() -> (w187:i32[])
        n104 = Greater Or Equal To 0?(x=w190) -> (x >= 0?=w191:bool)
        n105 = Array Size(array=w187) -> (size(s)=w188:i32)
        n106 = case shown="True" w191 {
          tunnel: w194 -> [w196 w202]
          tunnel: [w196 w201] -> w193
          tunnel: w190 -> [_ w200]
          tunnel: "StimChan" -> [_ w199]
          tunnel: w188 -> [_ w198]
          tunnel: w187 -> [_ w197]
          frame False {
          }
          frame True {
            n107 = case shown="2, Default" w198 {
              tunnel: w202 -> [w204 w219]
              tunnel: [w203 w216] -> w201
              tunnel: w200 -> [_ w214]
              tunnel: w199 -> [_ w213]
              tunnel: w197 -> [w205 _]
              frame 2, Default {
                n108 = for {
                  tunnel: w205 -> [w207] mode=indexing
                  shift-right: [w208] -> w203
                  shift-left: w204 -> [w209]
                  n109 = Index Array(array=w209, index=w207) -> (element=w210:T29)
                  n110 = invoke on="StimChan" class="Stimulus Channel (G3) (strict)" method="Get Multi.vi"("Value In"=w210) -> ("Value Out"=w206:T29)  [unwired: 4 in, 4 out]
                  n111 = Replace Array Subset(array=w209, new element=w206, index=w207) -> (w208:T29[])
                }
              }
              frame 1 {
                n112 = Replace Array Subset(array=w219, new element=w213, index=w214) -> (w217:T29[])
                n113 = for {
                  tunnel: w217 -> [w224] mode=indexing
                  tunnel: [w223] -> w218 mode=indexing
                  n114 = Unbundle By Name(w224) -> ("Name"=w223:string)
                }
                n115 = call "Array-Make Strings Unique.vi"("Strings"=w218) -> ("Unique Strings"=w215:string[])  [unwired: 4 in]
                n116 = for {
                  tunnel: w217 -> [w222] mode=indexing
                  tunnel: w215 -> [w221] mode=indexing
                  tunnel: [w220] -> w216 mode=indexing
                  n117 = Bundle By Name(cluster=w222, "Name"=w221) -> (w220:T29)
                }
                n118 = Index Array(array=w215, index=w214) -> (element=w212:string)
                n119 = Bundle By Name(cluster=w213, "Name"=w212) -> (w211:T28)
                n120 = property on="Channels" class="LstBox (strict)"("Item Names"=w215) -> ()  [unwired: 2 in, 2 out]
                n121 = local write "StimChan"(w211) -> ()
              }
            }
          }
        }
        n122 = Index Array(array=w187) -> (element=w189:i32)  [unwired: 1 in]
      }
    }
  }
  n123 = Destroy User Event(user event=w3) -> ()  [unwired: 1 in, 1 out]
  n124 = local write "StimChans In"(w1) -> ()
